vi "__uintComparisons.vi"(10 "Uint2 in":u8[](array[numeric])=[0], 11 "Uint1 in":u8[](array[numeric])=[0]) -> (0 "Timing comparison":u32, 2 "Uint1 != Uint2":bool, 3 "Uint1 = Uint2":bool, 4 "Uint1 <= Uint2":bool, 5 "Uint1 > Uint2":bool, 6 "Uint1 >= Uint2":bool, 7 "Uint1 < Uint2":bool)   [LabVIEW 2011, in "UintClass.lvclass"]
uses:
  UintClass.lvclass
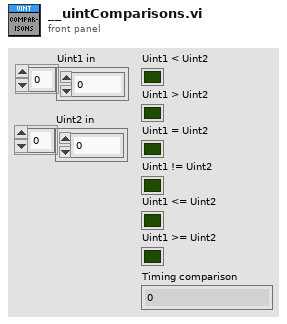
[diagram p1: front panel]
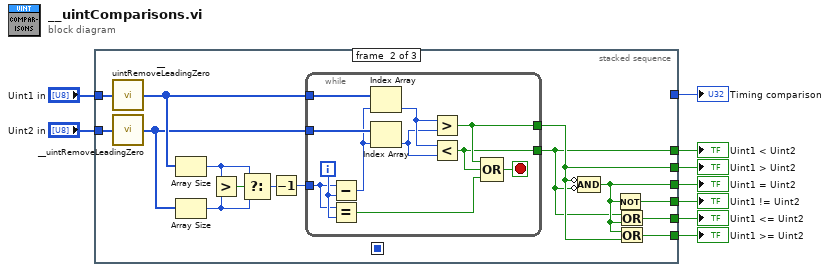
[diagram p0: block diagram]
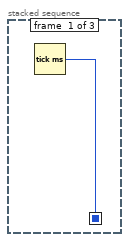
[diagram p2: hidden frame]
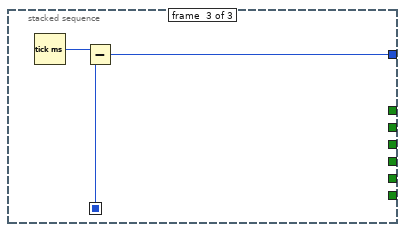
[diagram p3: hidden frame]
diagram:
  n1 = stacked-sequence {
    seq-local: [w10 _ _] -> [_ _ w38]
    tunnel: "Uint2 in" -> [_ w25 _]
    tunnel: "Uint1 in" -> [_ w24 _]
    tunnel: [_ w23 _] -> w7
    tunnel: [_ w22 _] -> w6
    tunnel: [_ w21 _] -> w5
    tunnel: [_ w20 _] -> w4
    tunnel: [_ w19 _] -> w3
    tunnel: [_ w18 _] -> w2
    tunnel: [_ _ w37] -> w1
    frame #0 {
      n2 = Tick Count (ms)() -> (millisecond timer value=w10:u32)
    }
    frame #1 {
      n3 = call "__uintRemoveLeadingZero.vi"("Uint in"=w24) -> ("Uint out"=w12:u8[])
      n4 = call "__uintRemoveLeadingZero.vi"("Uint in"=w25) -> ("Uint out"=w11:u8[])
      n5 = Array Size(array=w12) -> (size(s)=w15:i32)
      n6 = Array Size(array=w11) -> (size(s)=w16:i32)
      n7 = Greater?(x=w15, y=w16) -> (0:w14:bool)
      n8 = Select(t=w15, s=w14, f=w16) -> (s? t:f=w17:i32)
      n9 = Decrement(x=w17) -> (x-1=w13:i32)
      n10 = while {
        tunnel: w12 -> [w36]
        tunnel: w11 -> [w35]
        tunnel: [w30] -> w23
        tunnel: w13 -> [w33]
        tunnel: [w29] -> w20
        i -> [w34]
        stop <- w26 stop-if-true
        n11 = Subtract(x=w33, y=w34) -> (x-y=w27:i32)
        n12 = Equal?(x=w33, y=w34) -> (x = y?=w28:bool)
        n13 = Index Array(array=w36, index=w27) -> (element=w32:u8)
        n14 = Index Array(array=w35, index=w27) -> (element=w31:u8)
        n15 = Greater?(x=w32, y=w31) -> (0:w30:bool)
        n16 = Less?(x=w32, y=w31) -> (x < y?=w29:bool)
        n17 = Compound Arithmetic op=OR(w30, w29, w28) -> (w26:bool)
      }
      n18 = Compound Arithmetic op=AND(invert w23, invert w20) -> (w22:bool)
      n19 = Not(x=w22) -> (.not. x?=w18:bool)
      n20 = Or(x=w20, y=w22) -> (x .or. y?=w19:bool)
      n21 = Or(x=w22, y=w23) -> (x .or. y?=w21:bool)
    }
    frame #2 {
      n22 = Tick Count (ms)() -> (millisecond timer value=w39:u32)
      n23 = Subtract(x=w39, y=w38) -> (x-y=w37:u32)
    }
  }
  "Uint1 > Uint2" <- w7
  "Uint1 = Uint2" <- w6
  "Uint1 >= Uint2" <- w5
  "Uint1 < Uint2" <- w4
  "Uint1 <= Uint2" <- w3
  "Uint1 != Uint2" <- w2
  "Timing comparison" <- w1
